vi "FM_Rx_Template.vi"() -> ()   [LabVIEW 2013]
uses:
  <instrlib>/niUSRP/niUSRP Fetch Rx Data (CDB WDT).vi
  <vilib>/Analysis/NI_AALPro.lvlib
  <vilib>/Analysis/NI_AALBase.lvlib
  <vilib>/Analysis/3filter.llb/FIR Filter with I.C. (DBL).vi
  <vilib>/Analysis/3filter.llb/Butterworth Filter (DBL).vi
  <vilib>/measure/NI_MAPro.lvlib
  <vilib>/measure/maspectr.llb/FFT Power Spectrum and PSD for 1 Chan.vi
  <vilib>/Analysis/3filter.llb/Filter Passband Type.ctl
panel:
  in  "Peak Deviation":i64=200000
  out "Demodulated Signal":waveform(dbl)(graph)
  out "Demodulated Signal Spectrum":cluster{"f0":dbl, "df":dbl, "magnitude":dbl[]}(graph)
  in  "stop":bool
  out "Error Out":errorcluster
  in  "Number of Samples":i64=200000
  in  "Active Antenna":string(combo)="RX2"
  out "Actual Gain (dB)":dbl format="%#_6f"
  in  "Gain (dB)":dbl format="%#_6f"
  out "Actual Frequency":dbl=100000.0 format="%#_6p"
  in  "Carrier Frequency":dbl=915000000.0 format="%#_6p"
  out "Actual IQ Rate":dbl=100000.0 format="%#_6p"
  in  "IQ Rate":dbl=1000000.0 format="%#_6p"
  in  "Device Names":refnum<k15>="192.168.10.2"
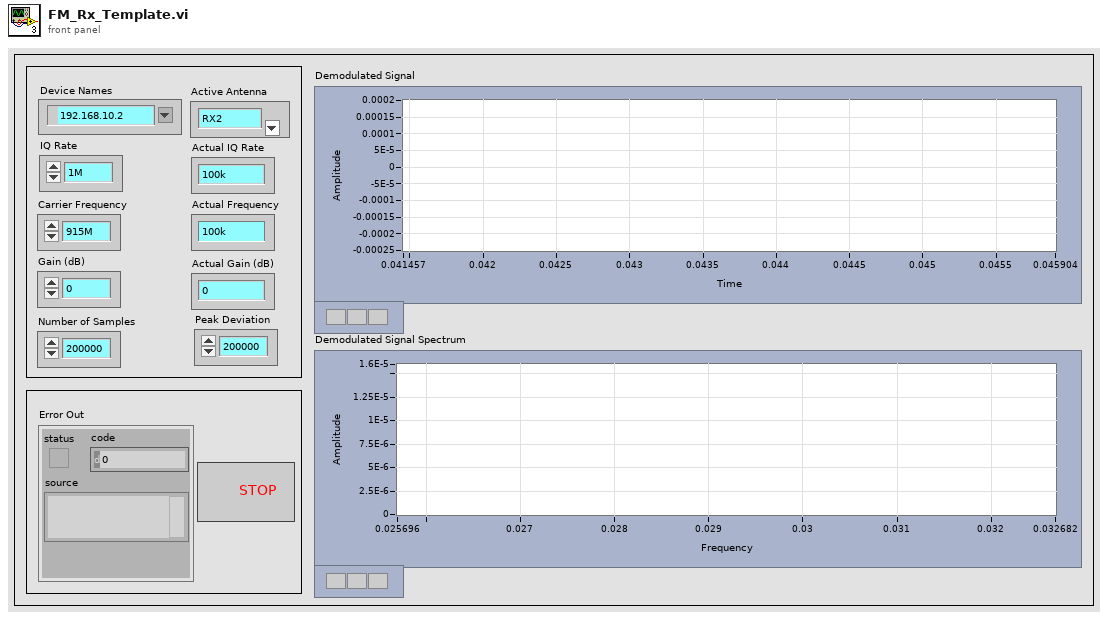
[diagram p1: front panel]
types:
  T1 = typedef "NI_AALBase.lvlib/Filter Passband Type.ctl" = enum32{"Lowpass", "Highpass", "Bandpass", "Bandstop"}
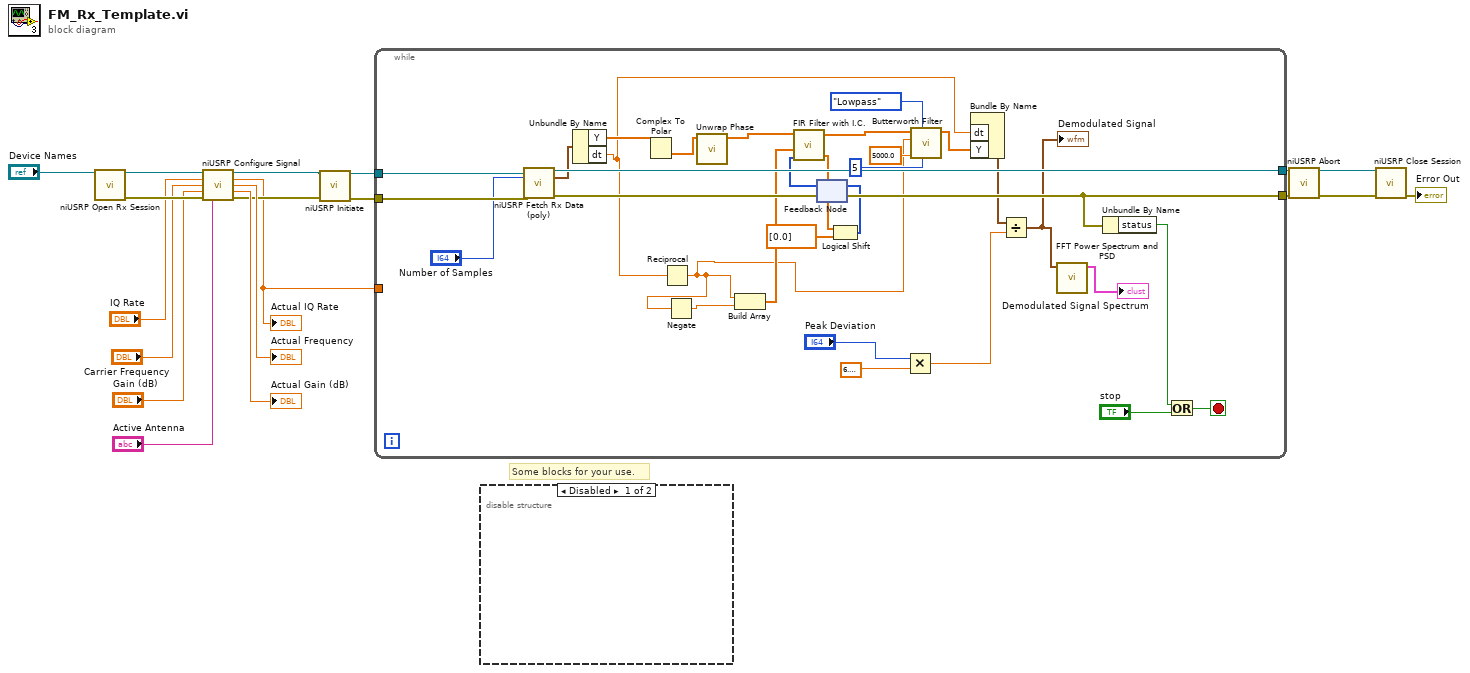
[diagram p0: block diagram]
diagram:
  # "Some blocks for your use."
  n1 = call <instrlib>:"niUSRP Open Rx Session.vi"("device names"="Device Names") -> ("session handle out"=w18:refnum<k15>, "error out"=w17:errorcluster)  [unwired: 13 in]
  n2 = call <instrlib>:"niUSRP Configure Signal.vi"("session handle"=w18, "IQ rate"="IQ Rate", "carrier frequency"="Carrier Frequency", "gain"="Gain (dB)", "error in (no error)"=w17, "active antenna"="Active Antenna") -> ("session handle out"=w11:refnum<k15>, "coerced IQ rate"=w1:dbl, "coerced carrier frequency"=→"Actual Frequency":dbl, "coerced gain"=→"Actual Gain (dB)":dbl, "error out"=w10:errorcluster)  [unwired: 5 in]
  "Actual IQ Rate" <- w1
  n3 = call <instrlib>:"niUSRP Initiate.vi"("session handle"=w11, "error in (no error)"=w10) -> ("session handle out"=w8:refnum<k15>, "error out"=w7:errorcluster)  [unwired: 12 in]
  n4 = while {
    tunnel: w8 -> [w50]
    tunnel: w7 -> [w49]
    tunnel: [w48] -> w6
    tunnel: [w44] -> w5
    tunnel: w1 -> [_]
    stop <- w47 stop-if-true
    n5 = call-poly <instrlib>:"niUSRP Fetch Rx Data (poly).vi"("session handle"=w50, "number of samples"="Number of Samples", "error in (no error)"=w49) -> ("session handle out"=w48:refnum<k15>, "data"=w20:waveform(cdb), "error out"=w44:errorcluster)  [unwired: 9 in, 1 out]
    n6 = Unbundle By Name(w20) -> ("Y"=w42:cdb[], "dt"=w21:dbl)
    n7 = Complex To Polar(r * e^(i*theta)=w42) -> (theta=w41:dbl[])  [unwired: 1 out]
    n8 = Reciprocal(x=w21) -> (1/x=w30:dbl)
    n9 = Negate(x=w30) -> (-x=w39:dbl)
    n10 = call <vilib>:"Unwrap Phase.vi"("Phase"=w41) -> ("Unwrapped Phase"=w40:dbl[])  [unwired: 9 in, 1 out]
    n11 = Build Array(w30, w39) -> (w38:dbl[])
    n12 = feedback #1() -> (w33:u32[])  [unwired: 1 in]
    n13 = call-poly <vilib>:"FIR Filter with I.C..vi"("Initial X Conditions"=w33, "FIR Coefficients"=w38, "X"=w40) -> ("Final X Conditions"=w36:dbl[], "Filtered X"=w37:dbl[])  [unwired: 5 in, 1 out]
    n14 = Logical Shift(y=w36, x=dbl[] [0.0]) -> (x << y=w34:u32[])
    n15 = feedback-in #1(w34) -> ()
    n16 = Multiply(x="Peak Deviation", y=6.283185307179586) -> (x*y=w26:dbl)
    n17 = call-poly <vilib>:"Butterworth Filter.vi"("order"=5, "filter type"=Filter_Passband_Type."Lowpass", "low cutoff freq: fl"=5000.0, "sampling freq: fs"=w30, "X"=w37) -> ("Filtered X"=w29:dbl[])  [unwired: 3 in, 1 out]
    n18 = Bundle By Name("dt"=w21, "Y"=w29) -> (w25:waveform(dbl))  [unwired: 1 in]
    n19 = Divide(x=w25, y=w26) -> (x/y=w23:waveform(dbl))
    "Demodulated Signal" <- w23
    n20 = call-poly <vilib>:"FFT Power Spectrum and PSD.vi"("time signal"=w23) -> ("Power Spectrum / PSD"=→"Demodulated Signal Spectrum":cluster{"f0":dbl, "df":dbl, "magnitude":dbl[]})  [unwired: 7 in, 3 out]
    n21 = Unbundle By Name(w44) -> ("status"=w46:bool)
    n22 = Or(x=w46, y="stop") -> (x .or. y?=w47:bool)
  }
  n23 = disable-structure shown="Disabled" {
    frame Disabled {
    }
    frame Enabled {
    }
  }
  n24 = call <instrlib>:"niUSRP Abort.vi"("session handle"=w6, "error in (no error)"=w5) -> ("session handle out"=w4:refnum<k15>, "error out"=w3:errorcluster)  [unwired: 12 in]
  n25 = call <instrlib>:"niUSRP Close Session.vi"("session handle"=w4, "error in (no error)"=w3) -> ("error out"=→"Error Out":errorcluster)  [unwired: 13 in]
